vi "Con_ETH_Names.vi"(7 "Active ETH":bool[](array[boolean]), 11 "ETH_Names":string[](array[string])) -> (2 "Status":bool[](array[boolean]), 3 "To connect":string[](array[string]))   [LabVIEW 2022 SP3]
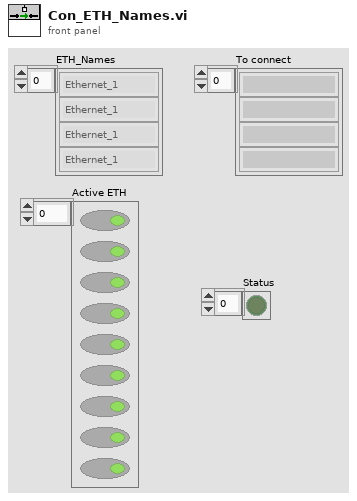
[diagram p1: front panel]
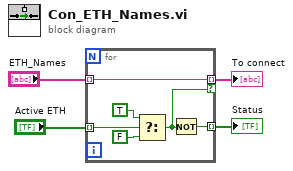
[diagram p0: block diagram]
diagram:
  n1 = for {
    tunnel: "ETH_Names" -> [w10] mode=indexing
    tunnel: [w10] -> w1 mode=indexing if=w7
    tunnel: [w6] -> w4 mode=indexing
    tunnel: "Active ETH" -> [w5] mode=indexing
    n2 = Select(t=TRUE, s=w5, f=FALSE) -> (s? t:f=w7:bool)
    n3 = Not(x=w7) -> (.not. x?=w6:bool)
  }
  "To connect" <- w1
  "Status" <- w4
